vi "Day 17 - Pyroclastic Flow.vi"() -> ()   [LabVIEW 2020, in "AoC 2022.lvlib"]
uses:
  AoC 2022.lvlib
  private/Sequence Analysis.ctl
  private/Pyroclastic Rock Shape.ctl
panel:
  in  "Calculate Height for #Rocks":u64[](array[numeric])=[2022, 1000000000000]
  out "Calculated Height":u64[](array[numeric])
  out "Sequence Analysis":T1
  out "#Rocks Settled":i32
  in  "#Rocks":i32=2022
  out "Height":u64
  in  "Auto Play Timer (ms)":i32=-1
  out "Current Action":string
  out "Push":string
  out "Current Rock":u32[][](array[colorbox])
  out "Chamber":u32[][](array[colorbox])
  out "Puzzle Part-2 Answer":dbl[](array[numeric]) format="%#_15f"
  in  "Puzzle Input":string=">>><<><>><<<>><>>><<<>>><<<><<<>><>><<>>"
  # "Press Ctrl+M & Enter the Puzzle Input and run the VI"
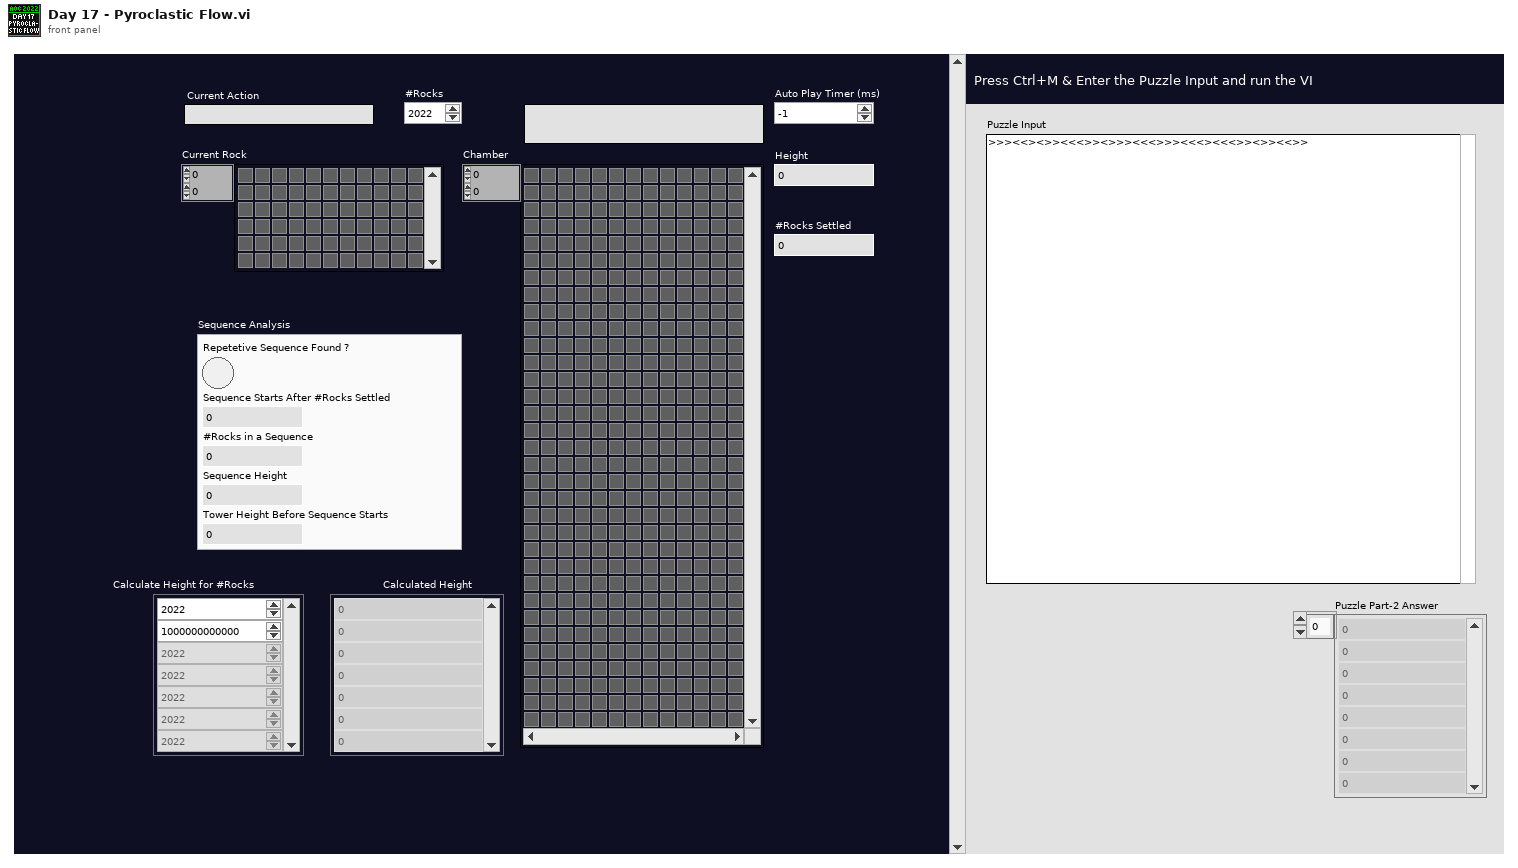
[diagram p1: front panel]
types:
  T1 = typedef "AoC 2022.lvlib/Sequence Analysis.ctl" = cluster{"Repetetive Sequence Found ?":bool, "Sequence Starts After #Rocks Settled":i32, "#Rocks in a Sequence":i32, "Sequence Height":u64, "Tower Height Before Sequence Starts":u64}
  T2 = typedef "AoC 2022.lvlib/Pyroclastic Rock Shape.ctl" = enum16{"_", "+", "_|", "|", "."}
  T3 = typedef "eventvkey.ctl" = enum16{"ASCII", "Enter", "Return", "Shift", "Ctrl", "Alt", "Cmd", "Opt", "Caps", "NumLock", "Clear", "Break", "Up", "Down", "Left", "Right", "Insert", "Delete", "Home", "End", "PageUp", "PageDown", "Escape", "Help", "Pause", "ScrollLock", "F1", "F2", "F3", "F4", "F5", "F6", "F7", "F8", "F9", "F10", "F11", "F12", "F13", "F14", "F15", "F16", "F17", "F18", "F19", "F20", "F21", "F22", "F23", "F24", "Play", "VolumeUp", "VolumeDown", "Mute", "Two Byte Char"}
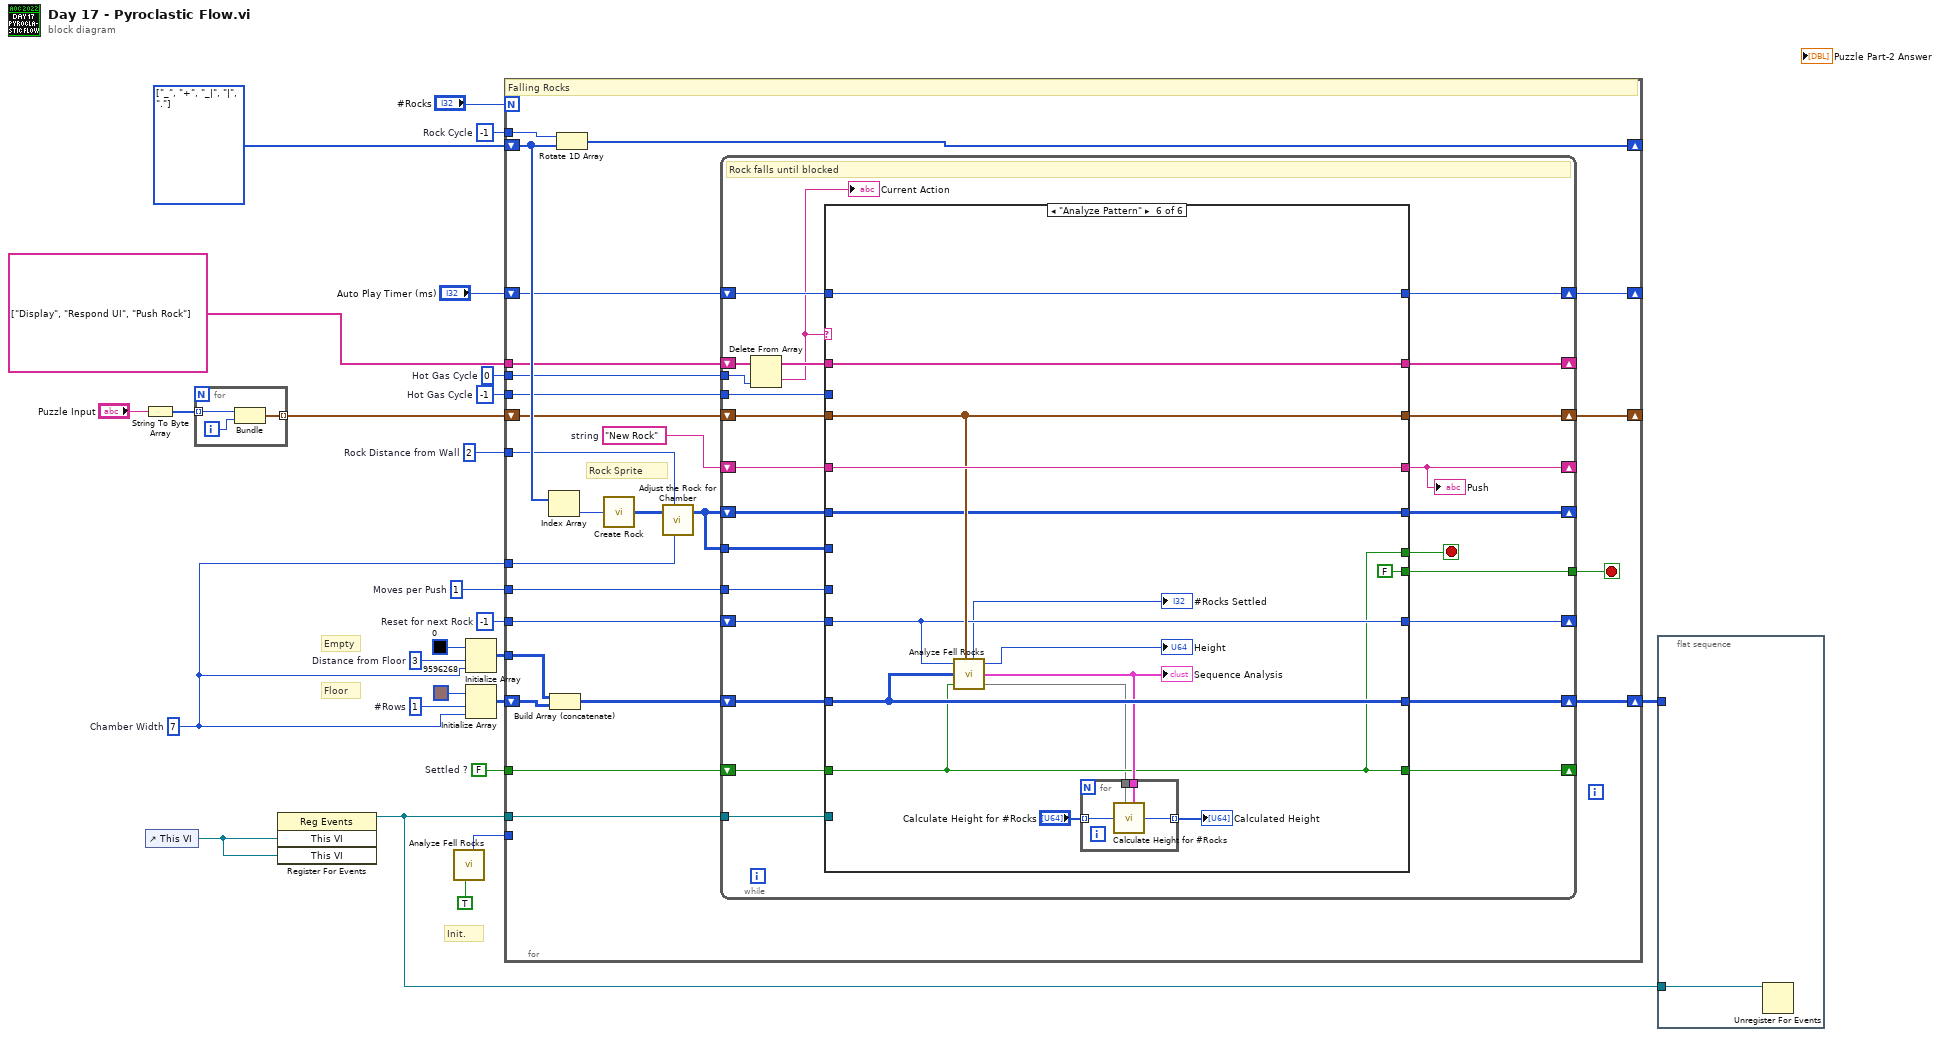
[diagram p0: block diagram]
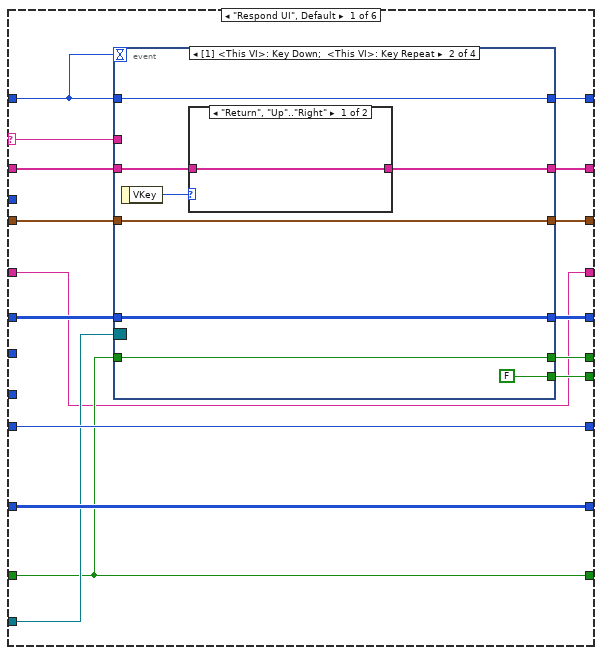
[diagram p2: hidden frame]
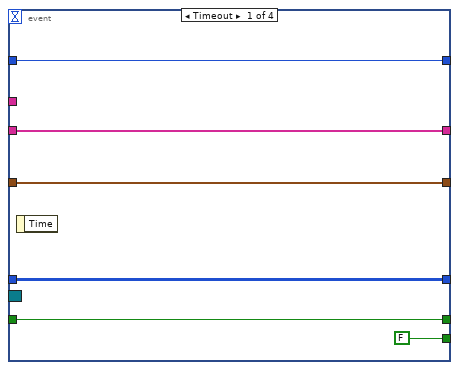
[diagram p3: hidden frame]
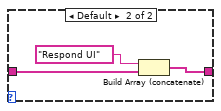
[diagram p4: hidden frame]
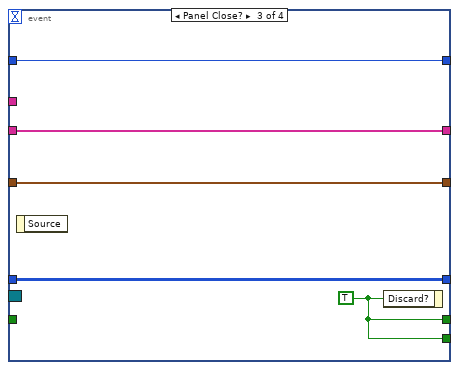
[diagram p5: hidden frame]
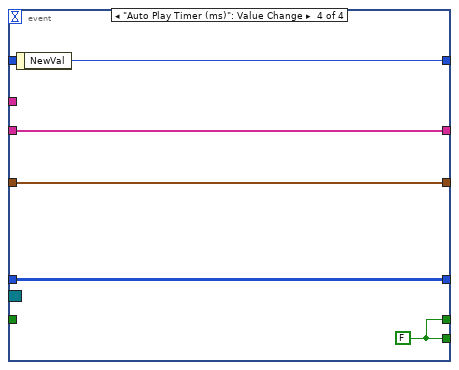
[diagram p6: hidden frame]
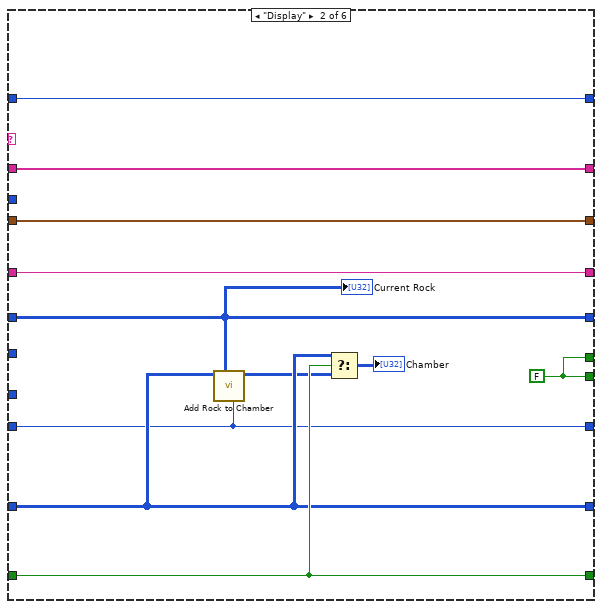
[diagram p7: hidden frame]
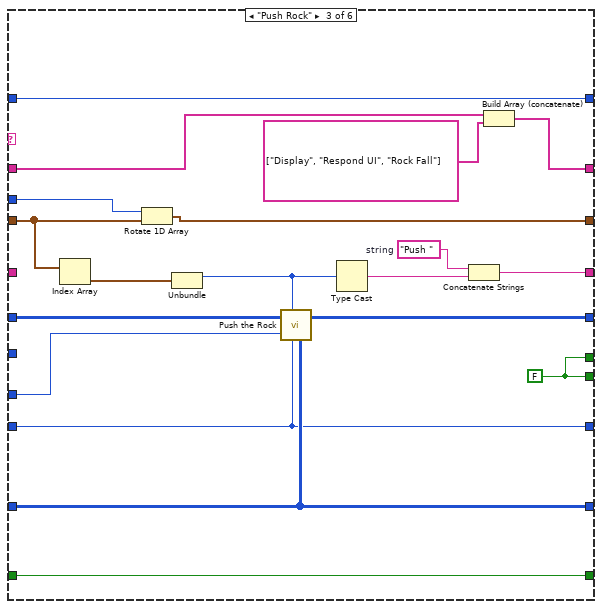
[diagram p8: hidden frame]
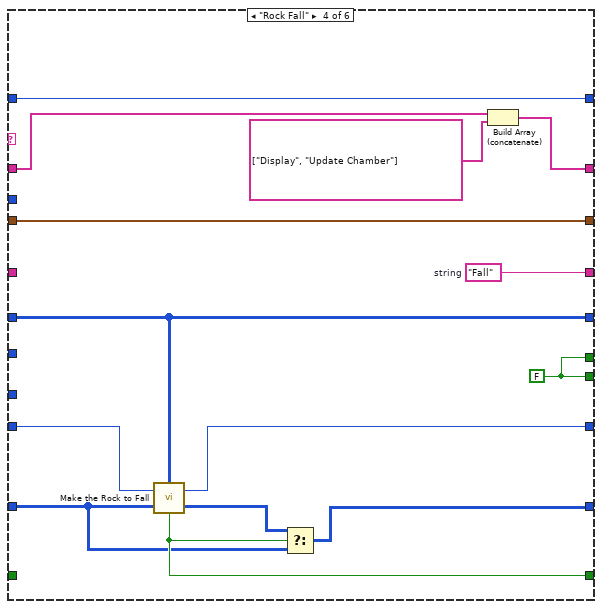
[diagram p9: hidden frame]
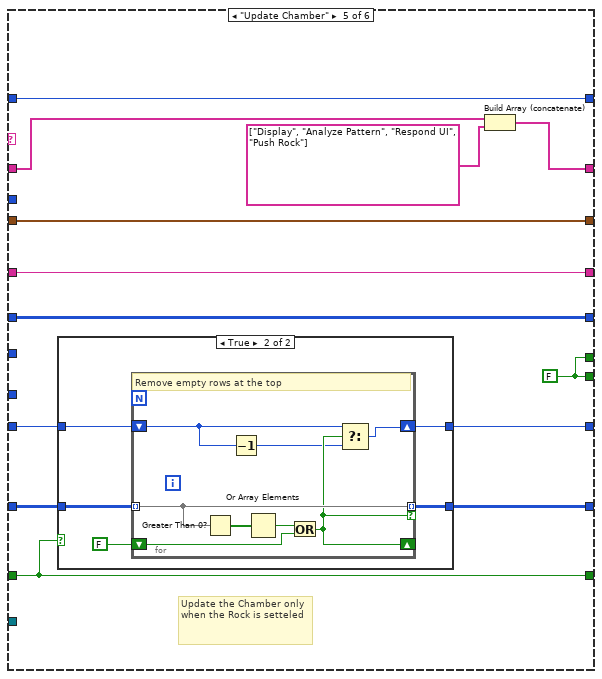
[diagram p10: hidden frame]
diagram:
  w7 = 0  # Hot Gas Cycle
  w12 = FALSE  # Settled ?
  w15 = -1  # Reset for next Rock
  w17 = 2  # Rock Distance from Wall
  w19 = -1  # Hot Gas Cycle
  w18 = 1  # Moves per Push
  w16 = 3  # Distance from Floor
  w22 = 1  # #Rows
  w14 = 7  # Chamber Width
  w24 = -1  # Rock Cycle
  w25 = T2[] [enum."_", enum."+", enum."_|", enum."|", enum."."] items=["_", "+", "_|", "|", "."]
  # "Empty"
  # "Init."
  # "Floor"
  n1 = String To Byte Array(string="Puzzle Input") -> (unsigned byte array=w3:u8[])
  n2 = control-ref of="This VI"() -> (w11:refnum<vi>)
  n3 = for {
    tunnel: w3 -> [w29] mode=indexing
    tunnel: [w27] -> w2 mode=indexing
    i -> [w28]
    n4 = Bundle(w29, w28) -> (w27:cluster{u8, i32})  [unwired: 1 in]
  }
  n5 = register-events(w11, w11) -> (reference out=w10:refnum<event-registration>)  [unwired: 2 in, 1 out]
  n6 = call "Analyze Fell Rocks.vi"("Initialize ? (F)"=TRUE) -> ("#Rocks Settled"=w1:i32)  [unwired: 5 in, 3 out]
  n7 = Initialize Array(u32 0, w16, w14) -> (w21:u32[][])
  n8 = Initialize Array(u32 9596268, w22, w14) -> (w23:u32[][])
  n9 = for {
    N: "#Rocks" -> [_]
    tunnel: w24 -> [w54]
    shift-right: [w53] -> _
    shift-left: w25 -> [w52]
    shift-right: [w31] -> w9
    shift-left: w23 -> [w50]
    tunnel: w21 -> [w49]
    shift-right: [w47] -> _
    shift-left: w2 -> [w48]
    tunnel: w19 -> [w46]
    tunnel: w18 -> [w45]
    tunnel: w14 -> [w43]
    tunnel: w17 -> [w42]
    tunnel: w15 -> [w41]
    shift-right: [w32] -> _
    shift-left: "Auto Play Timer (ms)" -> [w39]
    tunnel: w12 -> [w36]
    tunnel: w10 -> [w35]
    tunnel: string[] ["Display", "Respond UI", "Push Rock"] -> [w38]
    tunnel: w7 -> [w34]
    tunnel: w1 -> [_]
    stop <- w37 stop-if-true
    w33 = "New Rock"  # string
    # "Rock Sprite"
    # "Falling Rocks"
    n10 = Index Array(array=w52) -> (element=w51:T2)  [unwired: 1 in]
    n11 = Build Array (concatenate)(w49, w50) -> (w40:u32[][])
    n12 = Rotate 1D Array(1:w52, 2:w54) -> (0:w53:T2[])
    n13 = call "Create Rock.vi"("Pyroclastic Rock Shape"=w51) -> ("Rock"=w44:u32[][])  [unwired: 1 out]
    n14 = call "Adjust the Rock for Chamber.vi"("Chamber Width"=w43, "Rock in"=w44, "Rock Distance from Wall"=w42) -> ("Rock out"=w30:u32[][])  [unwired: 4 in]
    n15 = while {
      shift-right: [w56] -> w31
      shift-left: w40 -> [w71]
      shift-right: [w77] -> w47
      shift-left: w48 -> [w79]
      tunnel: w46 -> [w78]
      tunnel: w45 -> [w73]
      shift-right: [w69] -> _
      shift-left: w41 -> [w72]
      shift-right: [w70] -> _
      shift-left: w30 -> [w74]
      shift-right: [w75] -> w32
      shift-left: w39 -> [w76]
      shift-right: [w63] -> _
      shift-left: w38 -> [w62]
      tunnel: [w68] -> w37
      shift-right: [w65] -> _
      shift-left: w36 -> [w67]
      tunnel: w35 -> [w64]
      tunnel: w34 -> [w59]
      shift-right: [w58] -> _
      shift-left: w33 -> [w57]
      tunnel: w30 -> [w55]
      stop <- w66 stop-if-true
      # "Rock falls until blocked"
      n16 = Delete From Array(array=w62, index=w59) -> (deleted portion=w60:string, array with subset deleted=w61:string[])  [unwired: 1 in]
      "Current Action" <- w60
      n17 = case shown="\"Analyze Pattern\"" w60 {
        selector: w60 -> [w85 _ _ _ _ _]
        tunnel: w79 -> [w94 w133 w150 w166 w180 w205]
        tunnel: w78 -> [_ _ w153 _ _ _]
        tunnel: [w95 w133 w152 w166 w180 w205] -> w77
        tunnel: w76 -> [w92 w134 w151 w167 w179 w210]
        tunnel: [w93 w134 w151 w167 w179 w210] -> w75
        tunnel: [w91 w132 w139 w159 w173 w209] -> w63
        tunnel: w61 -> [w90 w132 w141 w160 w172 w209]
        tunnel: w74 -> [w88 w125 w149 w165 w175 w203]
        tunnel: w73 -> [_ _ w148 _ _ _]
        tunnel: w72 -> [w84 w124 w145 w164 w170 w204]
        tunnel: w71 -> [w83 w129 w146 w155 w178 w206]
        tunnel: [w89 w125 w147 w165 w175 w203] -> w70
        tunnel: [w83 w129 w146 w156 w177 w206] -> w56
        tunnel: [w84 w124 w145 w163 w169 w204] -> w69
        tunnel: [w87 w131 w144 w162 w176 w199] -> w66
        tunnel: [w86 w131 w144 w162 w176 FALSE] -> w68
        tunnel: w67 -> [w81 w130 w142 _ w168 w199]
        tunnel: [w81 w130 w142 w158 w168 w199] -> w65
        tunnel: w64 -> [w82 _ _ _ _ _]
        tunnel: [w80 w126 w137 w154 w171 w208] -> w58
        tunnel: w57 -> [w80 w126 _ _ w171 w208]
        tunnel: w55 -> [_ _ _ _ _ _]
        frame "Respond UI", Default {
          n18 = event shown="[1] <This VI>: Key Down;  <This VI>: Key Repeat" {
            selector: w82 -> [_ _ _ _]
            dyn-events: _ -> [_ _ _ _]
            timeout: w92 -> [_ _ _ _]
            tunnel: [w101 w109 w118 w123] -> w95
            tunnel: w94 -> [w101 w109 w118 w123]
            tunnel: [w100 w108 w115 w122] -> w93
            tunnel: w92 -> [w100 w108 w115 _]
            tunnel: [w97 w104 w114 w119] -> w91
            tunnel: w90 -> [w97 w107 w114 w119]
            tunnel: [w99 w106 w117 w121] -> w89
            tunnel: w88 -> [w99 w106 w117 w121]
            tunnel: [w96 w102 w116 w120] -> w87
            tunnel: [FALSE FALSE w116 w120] -> w86
            tunnel: w85 -> [_ _ _ _]
            tunnel: w81 -> [w96 w102 _ _]
            event Timeout {
              n19 = event-data() -> ()  [unwired: 1 in, 1 out]
            }
            event Key Down; Key Repeat {
              n20 = event-data() -> ("VKey"=w103:T3)  [unwired: 1 in]
              n21 = case shown="\"Return\", \"Up\"..\"Right\"" w103 {
                tunnel: w107 -> [w110 w113]
                tunnel: [w110 w112] -> w104
                frame "Return", "Up".."Right" {
                }
                frame Default {
                  n22 = Build Array (concatenate)("Respond UI" ("String"), w113) -> (w112:string[])
                }
              }
            }
            event Panel Close? {
              w116 = TRUE
              n23 = event-data() -> ()  [unwired: 1 in, 1 out]
              n24 = event-data("Discard?"=w116) -> ()  [unwired: 1 in, 1 out]
            }
            event "Auto Play Timer (ms)": Value Change {
              w120 = FALSE
              n25 = event-data() -> ("NewVal"=w122:i32)  [unwired: 1 in]
            }
          }
        }
        frame "Display" {
          w131 = FALSE
          n26 = call "Add Rock to Chamber.vi"("Rock Position in Chamber in"=w124, "Rock"=w125, "Chamber in"=w129) -> ("Chamber out"=w128:u32[][])  [unwired: 5 in, 1 out]
          n27 = Select(t=w129, s=w130, f=w128) -> (s? t:f=→"Chamber":u32[][])
          "Current Rock" <- w125
        }
        frame "Push Rock" {
          w136 = "Push "  # string
          w144 = FALSE
          n28 = Index Array(array=w150) -> (element=w143:cluster{u8, i32})  [unwired: 1 in]
          n29 = Rotate 1D Array(1:w150, 2:w153) -> (0:w152:cluster{u8, i32}[])
          n30 = Unbundle(w143) -> (w135:u8)  [unwired: 1 out]
          n31 = call "Push the Rock.vi"("Move #Units per Push"=w148, "Rock Position in Chamber in"=w145, "Chamber"=w146, "Rock in"=w149, "Push Direction"=w135) -> ("Rock out"=w147:u32[][])  [unwired: 2 in]
          n32 = Type Cast(x=w135) -> (*(type *) &x=w138:string)  [unwired: 1 in]
          n33 = Concatenate Strings(w136, w138) -> (w137:string)
          n34 = Build Array (concatenate)(w141, string[] ["Display", "Respond UI", "Rock Fall"]) -> (w139:string[])
        }
        frame "Rock Fall" {
          w154 = "Fall"  # string
          w162 = FALSE
          n35 = call "Make the Rock to Fall.vi"("Chamber in"=w155, "Rock Position in Chamber in"=w164, "Rock in"=w165) -> ("Consider Wall Boundary ? (T)"=w158:bool, "Chamber out"=w157:u32[][], "Rock Position in Chamber out"=w163:i32)
          n36 = Select(t=w157, s=w158, f=w155) -> (s? t:f=w156:u32[][])
          n37 = Build Array (concatenate)(w160, string[] ["Display", "Update Chamber"]) -> (w159:string[])
        }
        frame "Update Chamber" {
          w176 = FALSE
          # "Update the Chamber only when the Rock is setteled"
          n38 = case shown="True" w168 {
            tunnel: w178 -> [w181 w187]
            tunnel: [w181 w186] -> w177
            tunnel: w170 -> [w182 w185]
            tunnel: [w182 w184] -> w169
            frame False {
            }
            frame True {
              n39 = for {
                tunnel: [w195] -> w186 mode=indexing if=w191
                tunnel: w187 -> [w195] mode=indexing
                shift-right: [w191] -> _
                shift-left: FALSE -> [w194]
                shift-right: [w190] -> w184
                shift-left: w185 -> [w189]
                # "Remove empty rows at the top"
                n40 = Greater Than 0?(x=w195) -> (x > 0?=w192:bool[])
                n41 = Decrement(x=w189) -> (x-1=w188:i32)
                n42 = Or Array Elements(Boolean array=w192) -> (logical OR=w193:bool)
                n43 = Or(x=w193, y=w194) -> (x .or. y?=w191:bool)
                n44 = Select(t=w189, s=w191, f=w188) -> (s? t:f=w190:i32)
              }
            }
          }
          n45 = Build Array (concatenate)(w172, string[] ["Display", "Analyze Pattern", "Respond UI", "Push Rock"]) -> (w173:string[])
        }
        frame "Analyze Pattern" {
          n46 = call "Analyze Fell Rocks.vi"("Rock Position in Chamber in"=w204, "Push List"=w205, "Chamber"=w206, "Rock Settled ?"=w199) -> ("#Rocks Settled"=→"#Rocks Settled":i32, "Tower Height"=→"Height":u64, "Sequence Analysis"=w202:T1, "Tower Heights"=w197:map{i32, u64})  [unwired: 2 in]
          "Sequence Analysis" <- w202
          n47 = for {
            tunnel: w202 -> [w214]
            tunnel: [w213] -> w198 mode=indexing
            tunnel: w197 -> [w212]
            tunnel: "Calculate Height for #Rocks" -> [w211] mode=indexing
            n48 = call "Calculate Height for #Rocks.vi"("Calculate Height for #Rocks"=w211, "Tower Heights"=w212, "Sequence Analysis"=w214) -> ("Tower Height"=w213:u64)
          }
          "Calculated Height" <- w198
        }
      }
      "Push" <- w58
    }
  }
  n49 = flat-sequence {
    tunnel: w10 -> [w215]
    tunnel: w9 -> [_]
    frame #0 {
      n50 = Unregister For Events(event registration refnum=w215) -> ()  [unwired: 1 in, 1 out]
    }
  }
